vi "CRYASIOGetSamples.vi"(7 "Limit":i32=30000, 8 "Data Length":i32, 10 "error in (no error)":errorcluster) -> (0 "Buffer Amount":i32, 1 "pData":i32[](array[numeric]), 2 "nResult":u32, 3 "error out":errorcluster)   [LabVIEW 2013]
uses:
  CRY_ASIO.dll
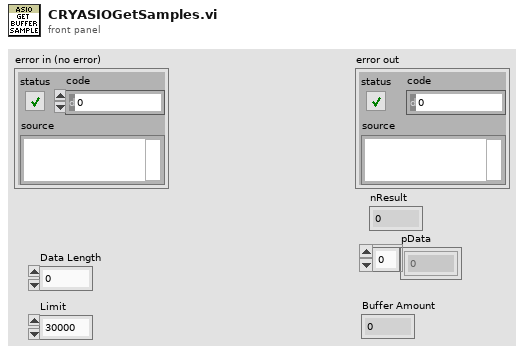
[diagram p1: front panel]
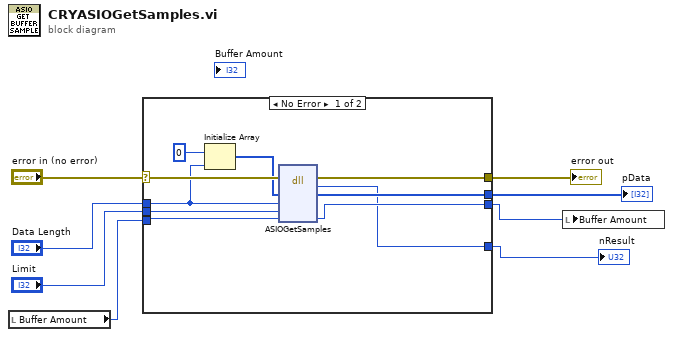
[diagram p0: block diagram]
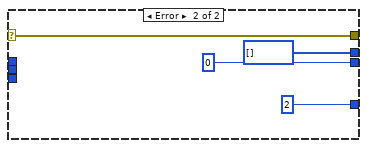
[diagram p2: hidden frame]
diagram:
  n1 = local read "Buffer Amount"() -> (w4:i32)
  n2 = case shown="No Error" "error in (no error)" {
    selector: "error in (no error)" -> [w18 w22]
    tunnel: [w17 w22] -> w7
    tunnel: "Data Length" -> [w12 _]
    tunnel: "Limit" -> [w16 _]
    tunnel: w4 -> [w15 _]
    tunnel: [w14 0 ("arg4")] -> w3
    tunnel: [w10 i32[] [] ("arg1")] -> w2
    tunnel: [w9 u32 2 ("return type")] -> w1
    frame No Error {
      n3 = Initialize Array(0, w12) -> (w11:i32[])
      n4 = dll-call lib="D:/LabView_Project/CRY6181/CRY_ASIO.dll" fn="ASIOGetSamples"(error in=w18, "arg1"=w11, "arg2"=w12, "arg3"=w16, "arg4"=w15) -> (error out=w17:errorcluster, "return type"=w9:u32, "arg1"=w10:i32[], "arg4"=w14:i32)  [unwired: 4 in, 1 out]
    }
    frame Error {
    }
  }
  "error out" <- w7
  "pData" <- w2
  "nResult" <- w1
  n5 = local write "Buffer Amount"(w3) -> ()
